vi "start list.vi"(8 "error in (no error)":errorcluster, 10 "time":dbl, 11 "identifier":string) -> (0 "error out":errorcluster, 3 "function return":u32)   [LabVIEW 2015, in "XGL_DPP.lvlib"]
doc: "EXTERN DECLSPEC unsigned int CALL_CONV start_list(const char* identifier, const double time);"
uses:
  XGL_DPP.lvlib
  D:/Scanning Software_Demokritos_2015_v6/libs/XGL_DPP.dll
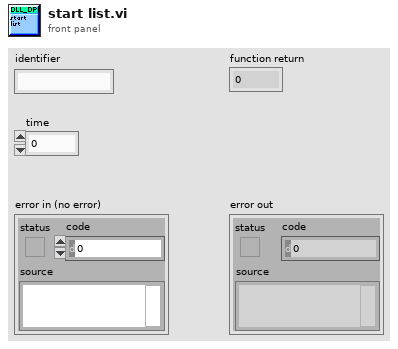
[diagram p1: front panel]
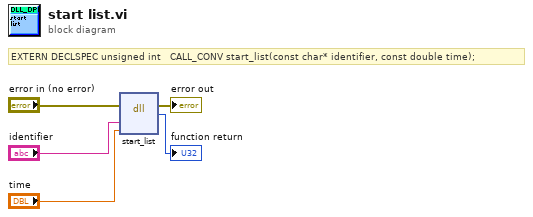
[diagram p0: block diagram]
diagram:
  # "EXTERN DECLSPEC unsigned int   CALL_CONV start_list(const char* identifier, const double time);"
  n1 = dll-call lib="D:/Scanning Software_Demokritos_2015_v6/libs/XGL_DPP.*" fn="start_list"(error in="error in (no error)", "identifier"="identifier", "time"="time") -> (error out=→"error out":errorcluster, "return type"=→"function return":u32)  [unwired: 4 in, 1 out]
